vi "SetLabelPosition__slk_mt.vi"(8 "error in (no error)":errorcluster, 10 "vi name":string, 11 "application reference":refnum<vi>) -> (0 "error out":errorcluster)   [LabVIEW 2015, in "Lazyboots Menu Tool.lvlib"]
doc: "This VI is the core of <b>Set Label Position</b> function, and will be called by corresponding menu launcher."
uses:
  <vilib>/SLK/Lazyboots Menu Tool/Library/Lazyboots Menu Tool.lvlib
  <vilib>/SLK/Lazyboots Menu Tool/Private/SetLabelPosition/TypeDef/TypeDef_SetLabelPositionState__slk_mt.ctl
  <vilib>/Utility/config.llb/NI_LVConfig.lvlib
panel:
  # "SetLabelPosition__slk_mt.vi\nThis VI is the core of <b>Set Label Position</b> function, and will be called by corresponding menu launcher.\n\nNOTICE -- YOU MUST LEAVE THIS NOTICE IN PLACE.\n\nCopyright (c) 2011, LIANG LIU Shawn.Liu.cn@gmail.com\nAll rights reserved.\n\nRedistribution and use in source and binary forms, with or without modification, are permitted provided that the following conditions are met:\n-Redistributions of source code must retain the above copyright notice, this list of conditions and the following disclaimer.\n-Redistributions in binary form must reproduce the above copyright notice, this list of conditions and the following disclaimer in the documentation and/or other materials provided with the distribution.\n-Neither the name of the eLp nor the names of its contributors may be used to endorse or promote products derived from this software without specific prior written permission.\n\nTHIS SOFTWARE IS PROVIDED BY THE COPYRIGHT HOLDERS AND CONTRIBUTORS \"AS IS\" AND ANY EXPRESS OR IMPLIED WARRANTIES, INCLUDING, BUT NOT LIMITED TO, THE IMPLIED WARRANTIES OF MERCHANTABILITY AND FITNESS FOR A PARTICULAR PURPOSE ARE DISCLAIMED. IN NO EVENT SHALL THE COPYRIGHT HOLDER OR CONTRIBUTORS BE LIABLE FOR ANY DIRECT, INDIRECT, INCIDENTAL, SPECIAL, EXEMPLARY, OR CONSEQUENTIAL DAMAGES (INCLUDING, BUT NOT LIMITED TO, PROCUREMENT OF SUBSTITUTE GOODS OR SERVICES; LOSS OF USE, DATA, OR PROFITS; OR BUSINESS INTERRUPTION) HOWEVER CAUSED AND ON ANY THEORY OF LIABILITY, WHETHER IN CONTRACT, STRICT LIABILITY, OR TORT (INCLUDING NEGLIGENCE OR OTHERWISE) ARISING IN ANY WAY OUT OF THE USE OF THIS SOFTWARE, EVEN IF ADVISED OF THE POSSIBILITY OF SUCH DAMAGE."
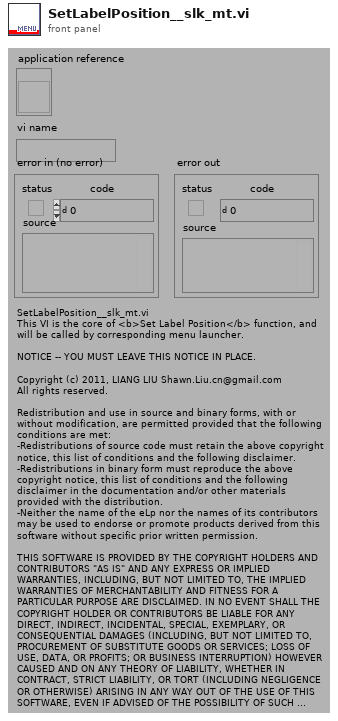
[diagram p1: front panel]
types:
  T1 = typedef "Lazyboots Menu Tool.lvlib/TypeDef_SetLabelPositionState__slk_mt.ctl" = enum16{"Read Configure", "Get Menu Launch VI", "Get Selected GObjects Refnums", "No Selection?", "Filter Refnums", "No Available?", "Undo.Start", "Set Position", "Deselect", "Message.No Selection", "Message.No Available", "Undo.End", "End"}
  T2 = typedef "NI_LVConfig.lvlib/Config Data RefNum.ctl" = refnum<k1>
  T3 = typedef "Lazyboots Menu Tool.lvlib/TypeDef_SetLabelPositionConfigure__slk_mt.ctl" = cluster{"Control Label Position":string, "Indicator Label Position":string, "Apply to All":bool}
  T4 = typedef "LVRectTypeDef.ctl" = cluster{"Left":i16, "Top":i16, "Right":i16, "Bottom":i16}
  T5 = typedef "LVBoundsTypeDef.ctl" = cluster{"Width":u32, "Height":u32}
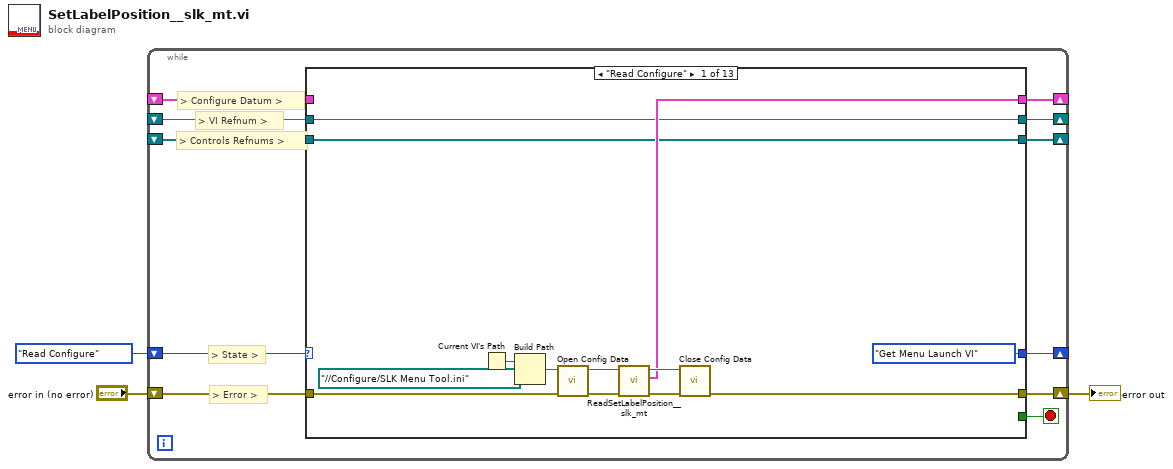
[diagram p0: block diagram]
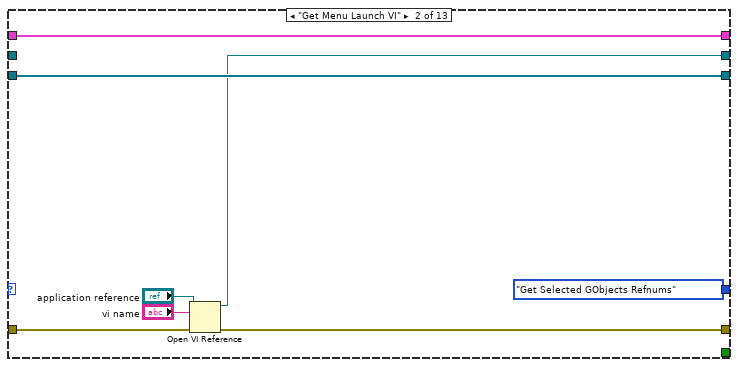
[diagram p2: hidden frame]
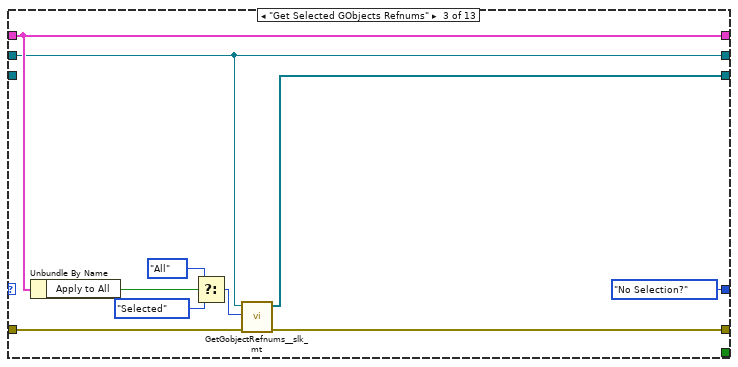
[diagram p3: hidden frame]
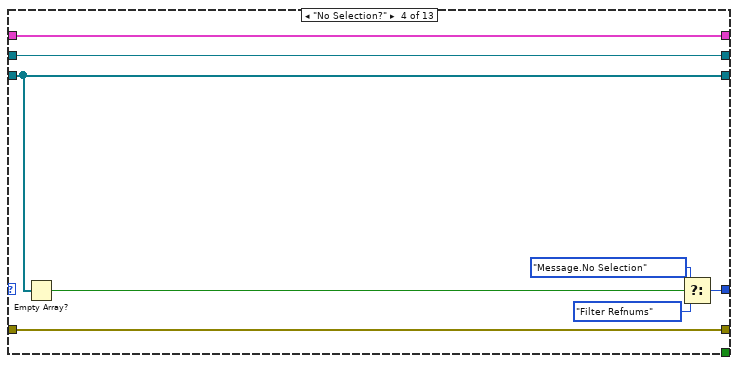
[diagram p4: hidden frame]
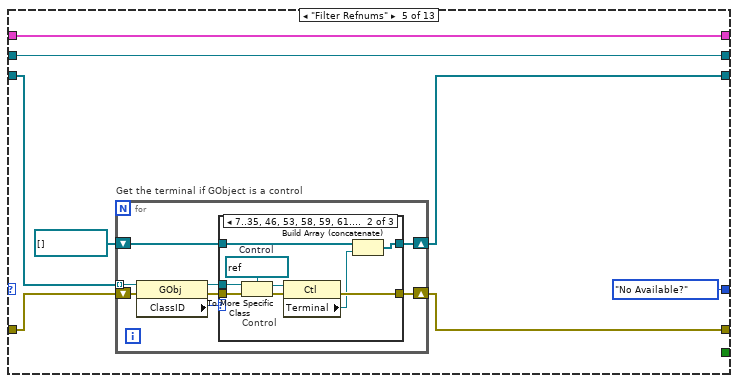
[diagram p5: hidden frame]
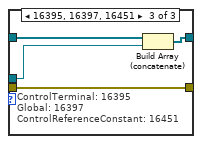
[diagram p7: hidden frame]
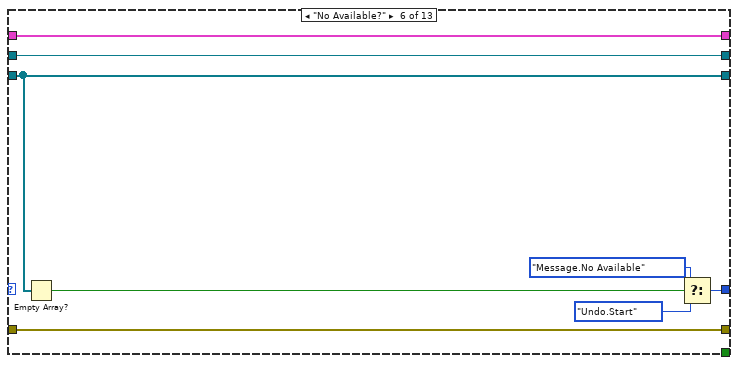
[diagram p8: hidden frame]
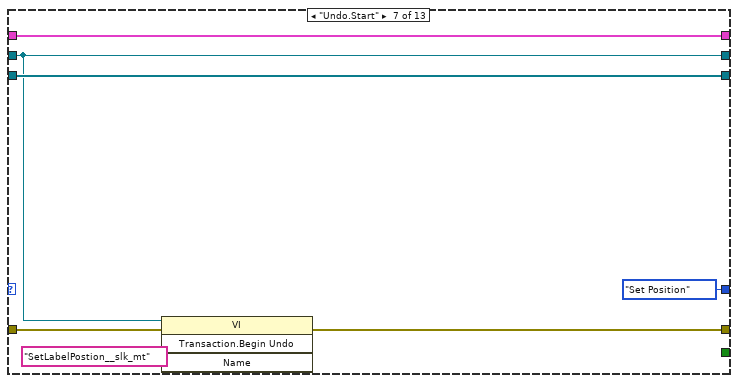
[diagram p9: hidden frame]
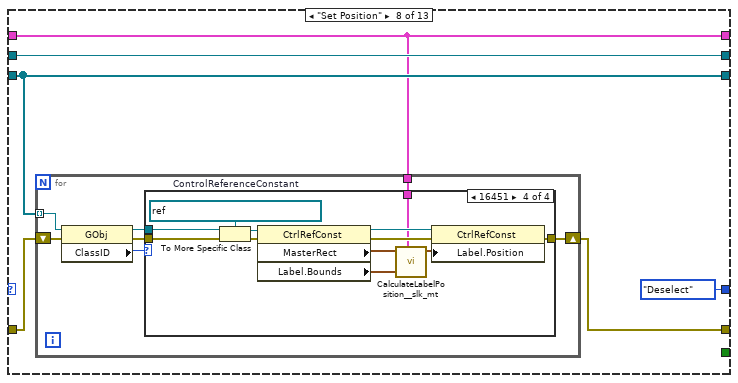
[diagram p10: hidden frame]
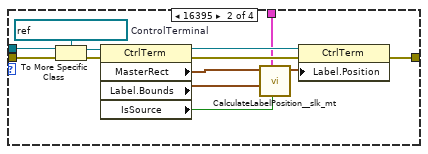
[diagram p12: hidden frame]
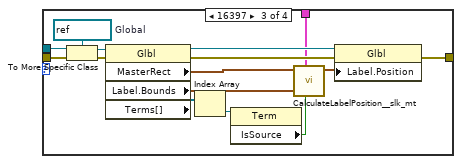
[diagram p13: hidden frame]
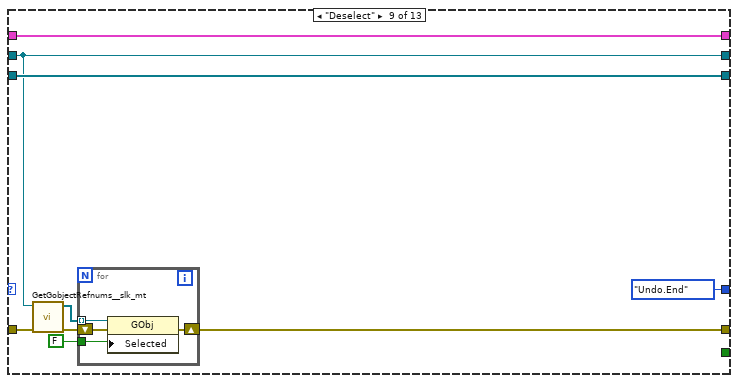
[diagram p14: hidden frame]
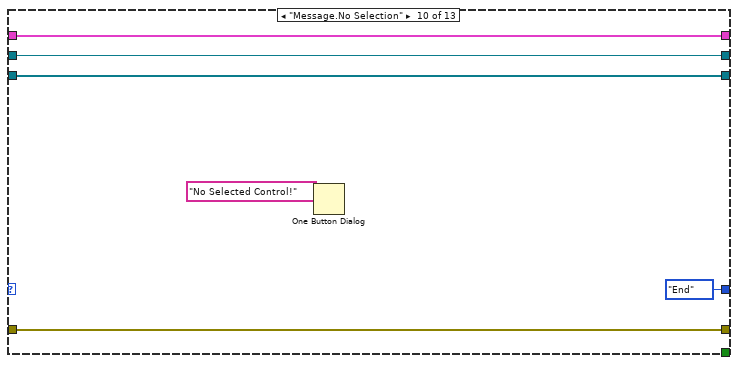
[diagram p15: hidden frame]
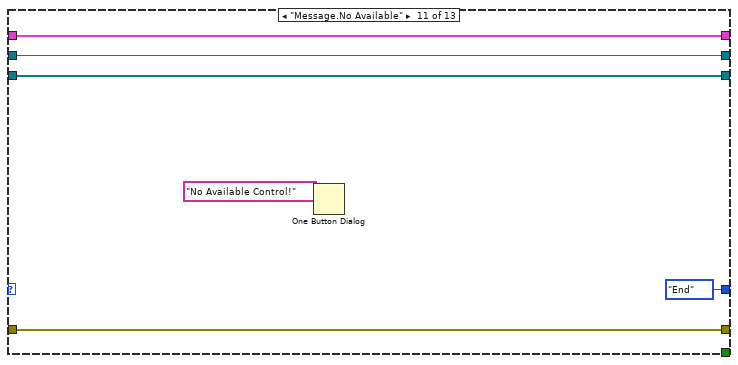
[diagram p16: hidden frame]
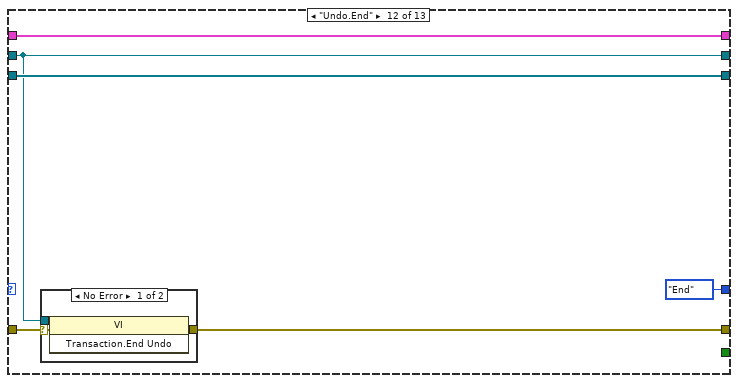
[diagram p17: hidden frame]
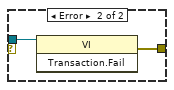
[diagram p18: hidden frame]
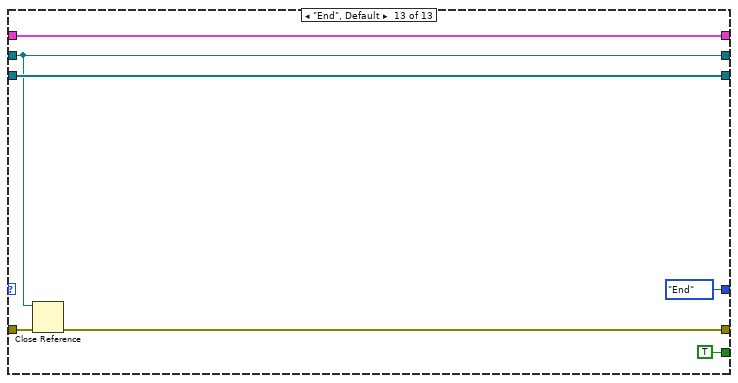
[diagram p19: hidden frame]
diagram:
  n1 = while {
    shift-right: [w11] -> _
    shift-left: TypeDef_SetLabelPositionState__slk_mt."Read Configure" ("State") -> [w14]
    shift-right: [w12] -> w1
    shift-left: "error in (no error)" -> [w13]
    shift-right: [w9] -> _
    shift-left: _ -> [w10]
    shift-right: [w7] -> _
    shift-left: _ -> [w8]
    shift-right: [w6] -> _
    shift-left: _ -> [w5]
    stop <- w4 stop-if-true
    # "> Controls Refnums >"
    # "> VI Refnum >"
    # "> Configure Datum >"
    # "> Error >"
    # "> State >"
    n2 = case shown="\"Read Configure\"" w14 {
      tunnel: w13 -> [w21 w35 w43 w51 w57 w90 w97 w102 w159 w169 w175 w181 w192]
      tunnel: [w19 w32 w42 w51 w56 w90 w96 w101 w154 w169 w175 w180 w191] -> w12
      tunnel: [TypeDef_SetLabelPositionState__slk_mt."Get Menu Launch VI" ("State") TypeDef_SetLabelPositionState__slk_mt."Get Selected GObjects Refnums" ("State") TypeDef_SetLabelPositionState__slk_mt."No Selection?" ("State") w47 TypeDef_SetLabelPositionState__slk_mt."No Available?" ("State") w86 TypeDef_SetLabelPositionState__slk_mt."Set Position" ("State") TypeDef_SetLabelPositionState__slk_mt."Deselect" ("State") TypeDef_SetLabelPositionState__slk_mt."Undo.End" ("State") TypeDef_SetLabelPositionState__slk_mt."End" ("State") TypeDef_SetLabelPositionState__slk_mt."End" ("State") TypeDef_SetLabelPositionState__slk_mt."End" ("State") TypeDef_SetLabelPositionState__slk_mt."End" ("State")] -> w11
      tunnel: w10 -> [_ w31 w44 w53 w61 w92 w99 w100 w160 w172 w178 w184 w195]
      tunnel: [w18 w31 w44 w53 w61 w92 w99 w100 w160 w172 w178 w184 w195] -> w9
      tunnel: w8 -> [w17 _ w41 w52 w60 w91 w95 w105 w158 w171 w177 w179 w190]
      tunnel: [w17 w30 w41 w52 w60 w91 w95 w105 w158 w171 w177 w179 w190] -> w7
      tunnel: [w16 w34 w40 w50 w54 w89 w98 w103 w161 w170 w176 w183 w196] -> w6
      tunnel: w5 -> [w16 w34 _ w50 w55 w89 w98 w103 w161 w170 w176 w183 w196]
      tunnel: [_ _ _ _ _ _ _ _ _ _ _ _ TRUE] -> w4
      frame "Read Configure" {
        n3 = Current VI's Path() -> (path=w23:path)
        n4 = Build Path(base path=w23, name or relative path=path "../../Configure/SLK Menu Tool.ini") -> (appended path=w22:path)
        n5 = call <vilib>:"Open Config Data.vi"("error in (no error)"=w21, "configuration file path"=w22) -> ("error out"=w26:errorcluster, "refnum"=w27:T2)  [unwired: 7 in, 1 out]
        n6 = call <vilib>:"ReadSetLabelPosition__slk_mt.vi"("error in (no error)"=w26, "refnum in"=w27) -> ("error out"=w25:errorcluster, "set label position configure"=w18:T3, "refnum out"=w24:T2)  [unwired: 7 in]
        n7 = call <vilib>:"Close Config Data.vi"("error in (no error)"=w25, "refnum"=w24) -> ("error out"=w19:errorcluster)  [unwired: 8 in, 1 out]
      }
      frame "Get Menu Launch VI" {
        n8 = Open VI Reference(application reference (local)="application reference", vi path="vi name", error in (no error)=w35) -> (vi reference=w30:refnum<vi>, error out=w32:errorcluster)  [unwired: 3 out]
      }
      frame "Get Selected GObjects Refnums" {
        n9 = Unbundle By Name(w44) -> ("Apply to All"=w37:bool)
        n10 = Select(t=enum16{"All", "Selected"}."All" ("from (Selected)"), s=w37, f=enum16{"All", "Selected"}."Selected" ("from (Selected)")) -> (s? t:f=w36:enum16{"All", "Selected"})
        n11 = call <vilib>:"GetGobjectRefnums__slk_mt.vi"("error in (no error)"=w43, "from (Selected)"=w36, "vi refnum in"=w41) -> ("error out"=w42:errorcluster, "generic objects refnums out"=w40:refnum<vi>[])  [unwired: 7 in]
      }
      frame "No Selection?" {
        n12 = Empty Array?(array=w50) -> (empty?=w46:bool)
        n13 = Select(t=TypeDef_SetLabelPositionState__slk_mt."Message.No Selection" ("State"), s=w46, f=TypeDef_SetLabelPositionState__slk_mt."Filter Refnums" ("State")) -> (s? t:f=w47:T1)
      }
      frame "Filter Refnums" {
        n14 = for "Get the terminal if GObject is a control" {
          tunnel: w55 -> [w69] mode=indexing
          shift-right: [w64] -> w56
          shift-left: w57 -> [w65]
          shift-right: [w62] -> w54
          shift-left: refnum<vi>[] [] -> [w63]
          n15 = property on="Property Node" class="GObj"(reference=w69, error in=w65) -> (reference out=w67:refnum<vi>, error out=w66:errorcluster, "ClassID"=w68:u32)
          n16 = case shown="7..35, 46, 53, 58, 59, 61..66, 68, 102" w68 {
            tunnel: w67 -> [_ w78 w81]
            tunnel: w66 -> [w70 w75 w82]
            tunnel: [w70 w73 w82] -> w64
            tunnel: w63 -> [w71 w80 w84]
            tunnel: [w71 w79 w83] -> w62
            frame Default {
            }
            frame 7..35, 46, 53, 58, 59, 61..66, 68, 102 {
              w74 = refnum<vi> refnum  # Control
              # "Control"
              n17 = To More Specific Class(target class=w74, reference=w78, error in=w75) -> (specific class reference=w77:refnum<vi>, error out=w76:errorcluster)
              n18 = property on="Property Node" class="Ctl"(reference=w77, error in=w76) -> (error out=w73:errorcluster, "Terminal"=w72:refnum<vi>)  [unwired: 1 out]
              n19 = Build Array (concatenate)(w80, w72) -> (w79:refnum<vi>[])
            }
            frame 16395, 16397, 16451 {
              # "ControlTerminal: 16395\nGlobal: 16397\nControlReferenceConstant: 16451"
              n20 = Build Array (concatenate)(w84, w81) -> (w83:refnum<vi>[])
            }
          }
        }
      }
      frame "No Available?" {
        n21 = Empty Array?(array=w89) -> (empty?=w85:bool)
        n22 = Select(t=TypeDef_SetLabelPositionState__slk_mt."Message.No Available" ("State"), s=w85, f=TypeDef_SetLabelPositionState__slk_mt."Undo.Start" ("State")) -> (s? t:f=w86:T1)
      }
      frame "Undo.Start" {
        n23 = invoke class="VI" method="Transaction.Begin Undo"(reference=w95, error in=w97, "Name"="SetLabelPostion__slk_mt") -> (error out=w96:errorcluster)  [unwired: 1 in, 3 out]
      }
      frame "Set Position" {
        n24 = for {
          shift-right: [w112] -> w101
          shift-left: w102 -> [w109]
          tunnel: w103 -> [w107] mode=indexing
          tunnel: w100 -> [w106]
          n25 = property class="GObj"(reference=w107, error in=w109) -> (reference out=w111:refnum<vi>, error out=w108:errorcluster, "ClassID"=w110:u32)
          n26 = case shown="16451" w110 {
            tunnel: w111 -> [_ w126 w141 w153]
            tunnel: [w113 w115 w128 w143] -> w112
            tunnel: w108 -> [w113 w120 w135 w147]
            tunnel: w106 -> [_ w114 w127 w142]
            frame Default {
            }
            frame 16395 {
              w123 = refnum<vi> refnum  # ControlTerminal
              n27 = To More Specific Class(target class=w123, reference=w126, error in=w120) -> (specific class reference=w125:refnum<vi>, error out=w124:errorcluster)
              n28 = property on="Property Node" class="CtrlTerm"(reference=w125, error in=w124) -> (reference out=w122:refnum<vi>, error out=w121:errorcluster, "MasterRect"=w119:T4, "Label.Bounds"=w118:T5, "IsSource"=w116:bool)
              n29 = call <vilib>:"CalculateLabelPosition__slk_mt.vi"("control? (t)"=w116, "set label position configure"=w114, "label bounds"=w118, "master bounds rectangle"=w119) -> ("label position"=w117:cluster{"Left":i32, "Top":i32})  [unwired: 7 in]
              n30 = property on="Property Node" class="CtrlTerm"(reference=w122, error in=w121, "Label.Position"=w117) -> (error out=w115:errorcluster)  [unwired: 1 out]
            }
            frame 16397 {
              w138 = refnum<vi> refnum  # Global
              n31 = To More Specific Class(target class=w138, reference=w141, error in=w135) -> (specific class reference=w140:refnum<vi>, error out=w139:errorcluster)
              n32 = property on="Property Node" class="Glbl"(reference=w140, error in=w139) -> (reference out=w137:refnum<vi>, error out=w136:errorcluster, "MasterRect"=w132:T4, "Label.Bounds"=w131:T5, "Terms[]"=w134:refnum<vi>[])
              n33 = Index Array(array=w134) -> (element=w130:refnum<vi>)  [unwired: 1 in]
              n34 = property on="Property Node" class="Term"(reference=w130) -> ("IsSource"=w129:bool)  [unwired: 1 in, 2 out]
              n35 = call <vilib>:"CalculateLabelPosition__slk_mt.vi"("control? (t)"=w129, "set label position configure"=w127, "label bounds"=w131, "master bounds rectangle"=w132) -> ("label position"=w133:cluster{"Left":i32, "Top":i32})  [unwired: 7 in]
              n36 = property on="Property Node" class="Glbl"(reference=w137, error in=w136, "Label.Position"=w133) -> (error out=w128:errorcluster)  [unwired: 1 out]
            }
            frame 16451 {
              w150 = refnum<vi> refnum  # ControlReferenceConstant
              n37 = To More Specific Class(target class=w150, reference=w153, error in=w147) -> (specific class reference=w152:refnum<vi>, error out=w151:errorcluster)
              n38 = property on="Property Node" class="CtrlRefConst"(reference=w152, error in=w151) -> (reference out=w149:refnum<vi>, error out=w148:errorcluster, "MasterRect"=w145:T4, "Label.Bounds"=w144:T5)
              n39 = call <vilib>:"CalculateLabelPosition__slk_mt.vi"("set label position configure"=w142, "label bounds"=w144, "master bounds rectangle"=w145) -> ("label position"=w146:cluster{"Left":i32, "Top":i32})  [unwired: 8 in]
              n40 = property on="Property Node" class="CtrlRefConst"(reference=w149, error in=w148, "Label.Position"=w146) -> (error out=w143:errorcluster)  [unwired: 1 out]
            }
          }
        }
      }
      frame "Deselect" {
        n41 = call <vilib>:"GetGobjectRefnums__slk_mt.vi"("error in (no error)"=w159, "vi refnum in"=w158) -> ("error out"=w157:errorcluster, "generic objects refnums out"=w156:refnum<vi>[])  [unwired: 8 in]
        n42 = for {
          shift-right: [w166] -> w154
          shift-left: w157 -> [w165]
          tunnel: w156 -> [w164] mode=indexing
          tunnel: FALSE -> [w163]
          n43 = property class="GObj"(reference=w164, error in=w165, "Selected"=w163) -> (error out=w166:errorcluster)  [unwired: 1 out]
        }
      }
      frame "Message.No Selection" {
        n44 = One Button Dialog(message="No Selected Control!") -> ()  [unwired: 2 out]
      }
      frame "Message.No Available" {
        n45 = One Button Dialog(message="No Available Control!") -> ()  [unwired: 2 out]
      }
      frame "Undo.End" {
        n46 = case shown="No Error" w181 {
          selector: w181 -> [w186 _]
          tunnel: w179 -> [w187 w189]
          tunnel: [w185 w188] -> w180
          frame No Error {
            n47 = invoke class="VI" method="Transaction.End Undo"(reference=w187, error in=w186) -> (error out=w185:errorcluster)  [unwired: 1 in, 2 out]
          }
          frame Error {
            n48 = invoke class="VI" method="Transaction.Fail"(reference=w189) -> (error out=w188:errorcluster)  [unwired: 2 in, 2 out]
          }
        }
      }
      frame "End", Default {
        n49 = Close Reference(reference=w190, error in (no error)=w192) -> (error out=w191:errorcluster)
      }
    }
  }
  "error out" <- w1
